vi "Conv_BIN2BCD_SubVI.vi"(4 "W":bool, 5 "X":bool, 6 "Y":bool, 7 "Z":bool) -> (0 "A":bool, 1 "B":bool, 2 "C":bool, 3 "D":bool)   [LabVIEW 2016]
doc: "Este SubVi nos entrega a la salida una decodificación BCD para una entrada binaria (4 bits mas significativos)."
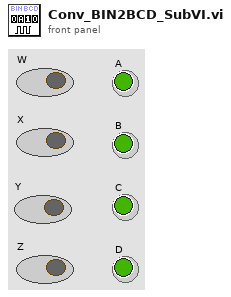
[diagram p1: front panel]
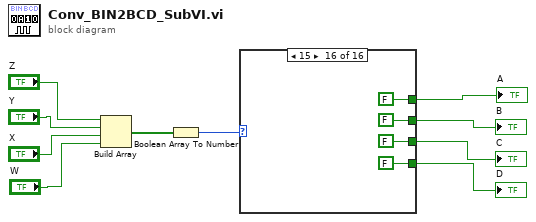
[diagram p0: block diagram]
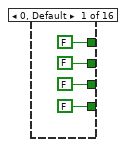
[diagram p2: hidden frame]
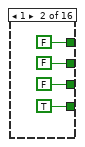
[diagram p3: hidden frame]
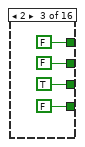
[diagram p4: hidden frame]
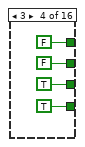
[diagram p5: hidden frame]
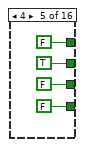
[diagram p6: hidden frame]
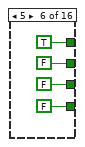
[diagram p7: hidden frame]
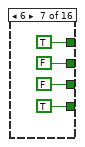
[diagram p8: hidden frame]
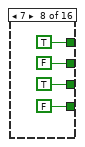
[diagram p9: hidden frame]
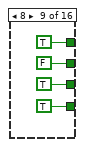
[diagram p10: hidden frame]
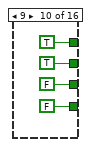
[diagram p11: hidden frame]
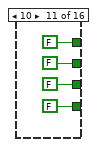
[diagram p12: hidden frame]
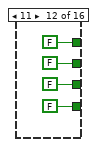
[diagram p13: hidden frame]
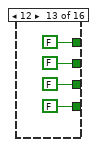
[diagram p14: hidden frame]
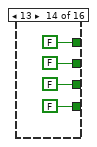
[diagram p15: hidden frame]
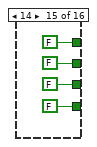
[diagram p16: hidden frame]
diagram:
  n1 = Build Array("Z", "Y", "X", "W") -> (w5:bool[])
  n2 = Boolean Array To Number(Boolean array=w5) -> (number=w6:u32)
  n3 = case shown="15" w6 {
    tunnel: [FALSE FALSE FALSE FALSE FALSE TRUE TRUE TRUE TRUE TRUE FALSE FALSE FALSE FALSE FALSE FALSE] -> w8
    tunnel: [FALSE FALSE FALSE FALSE TRUE FALSE FALSE FALSE FALSE TRUE FALSE FALSE FALSE FALSE FALSE FALSE] -> w7
    tunnel: [FALSE FALSE TRUE TRUE FALSE FALSE FALSE TRUE TRUE FALSE FALSE FALSE FALSE FALSE FALSE FALSE] -> w9
    tunnel: [FALSE TRUE FALSE TRUE FALSE FALSE TRUE FALSE TRUE FALSE FALSE FALSE FALSE FALSE FALSE FALSE] -> w10
    frame 0, Default {
    }
    frame 1 {
    }
    frame 2 {
    }
    frame 3 {
    }
    frame 4 {
    }
    frame 5 {
    }
    frame 6 {
    }
    frame 7 {
    }
    frame 8 {
    }
    frame 9 {
    }
    frame 10 {
    }
    frame 11 {
    }
    frame 12 {
    }
    frame 13 {
    }
    frame 14 {
    }
    frame 15 {
    }
  }
  "D" <- w10
  "C" <- w9
  "A" <- w8
  "B" <- w7
